vi "Animacion2.vi"() -> ()   [LabVIEW 2017]
uses:
  <vilib>/picture/picture.llb/Draw True-Color Pixmap.vi
panel:
  in  "Donde?":cluster{"x":i16, "y":i16}
  out "Mundo":picture
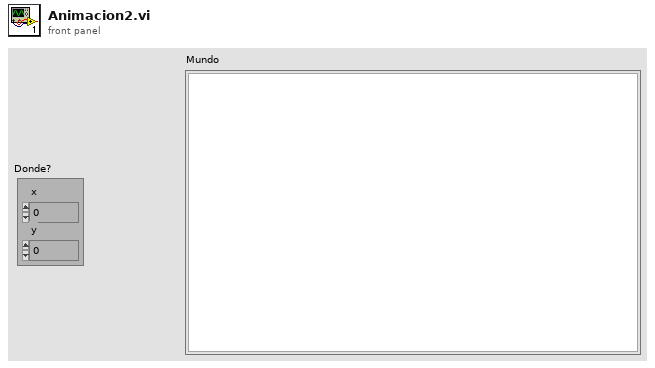
[diagram p1: front panel]
types:
  T1 = typedef "imagedata.ctl" = cluster{"image type":i32, "image depth":i32, "image":u8[], "mask":u8[], "colors":u32[], "Rectangle":cluster{"left":i16, "top":i16, "right":i16, "bottom":i16}}
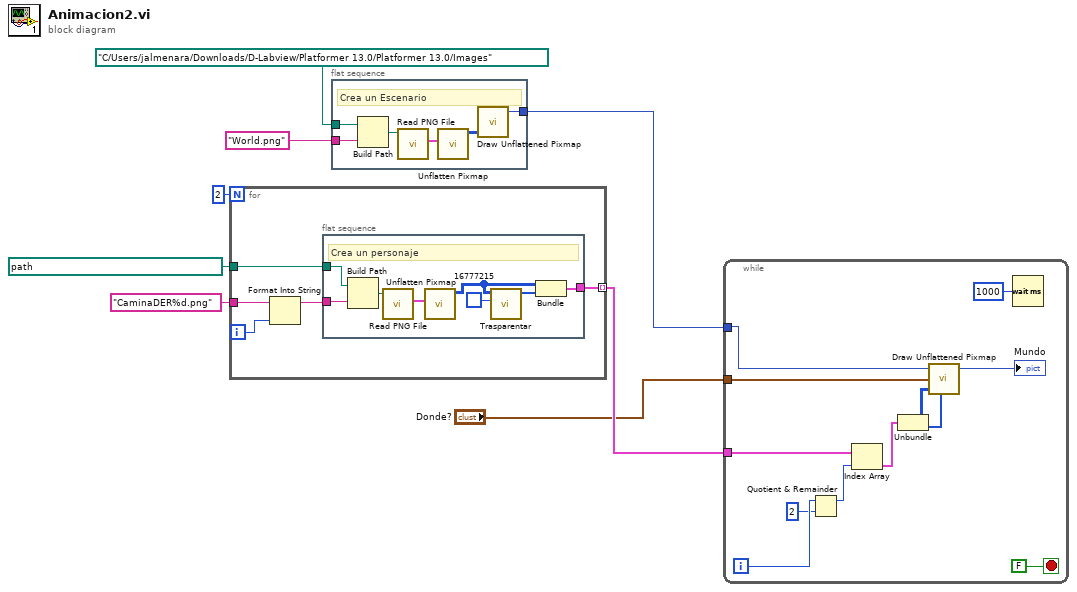
[diagram p0: block diagram]
diagram:
  n1 = for {
    N: 2 -> [_]
    tunnel: [w13] -> w5 mode=indexing
    tunnel: path "F:/Prog/LabVIEW/Pruebas/Animación" ("path to PNG file") -> [w10]
    tunnel: "CaminaDER%d.png" ("format string") -> [w9]
    i -> [w12]
    n2 = Format Into String(format string=w9, w12) -> (resulting string=w11:string)  [unwired: 2 in, 1 out]
    n3 = flat-sequence {
      tunnel: w11 -> [w21]
      tunnel: [w15] -> w13
      tunnel: w10 -> [w14]
      frame #0 {
        # "Crea un personaje"
        n4 = Build Path(base path=w14, name or relative path=w21) -> (appended path=w20:path)
        n5 = call <vilib>:"Read PNG File.vi"("path to PNG file"=w20) -> ("image data"=w19:T1)  [unwired: 8 in, 2 out]
        n6 = call <vilib>:"Unflatten Pixmap.vi"("image data"=w19) -> ("24-bit pixmap"=w17:u32[][])  [unwired: 4 in, 6 out]
        n7 = call "Trasparentar.vi"("Background Color"=u32 16777215, "24-bit pixmap"=w17) -> ("Mask"=w16:u8[])  [unwired: 9 in]
        n8 = Bundle("24-bit pixmap"=w17, "Mask"=w16) -> (w15:cluster{"24-bit pixmap":u32[][], "Mask":u8[]})  [unwired: 1 in]
      }
    }
  }
  n9 = flat-sequence {
    tunnel: "World.png" ("format string") -> [w26]
    tunnel: path "C:/Users/jalmenara/Downloads/D-Labview/Platformer 13.0/Platformer 13.0/Images" ("path to PNG file") -> [w25]
    tunnel: [w22] -> w3
    frame #0 {
      # "Crea un Escenario"
      n10 = Build Path(base path=w25, name or relative path=w26) -> (appended path=w24:path)
      n11 = call <vilib>:"Read PNG File.vi"("path to PNG file"=w24) -> ("image data"=w27:T1)  [unwired: 8 in, 2 out]
      n12 = call <vilib>:"Unflatten Pixmap.vi"("image data"=w27) -> ("24-bit pixmap"=w23:u32[][])  [unwired: 4 in, 6 out]
      n13 = call-poly <vilib>:"Draw Unflattened Pixmap.vi"("data (RGB format)"=w23) -> ("new picture"=w22:picture)  [unwired: 8 in]
    }
  }
  n14 = while {
    tunnel: w5 -> [w36]
    tunnel: "Donde?" -> [w32]
    tunnel: w3 -> [w28]
    i -> [w39]
    stop <- FALSE stop-if-true
    n15 = Quotient & Remainder(x=w39, y=2) -> (x-y*floor(x/y)=w37:i32)  [unwired: 1 out]
    n16 = Index Array(array=w36, index=w37) -> (element=w35:cluster{"24-bit pixmap":u32[][], "Mask":u8[]})
    n17 = Unbundle(w35) -> ("24-bit pixmap"=w34:u32[][], "Mask"=w33:u8[])
    n18 = call-poly <vilib>:"Draw Unflattened Pixmap.vi"("picture"=w28, "top left point(0, 0)"=w32, "data (RGB format)"=w34, "mask"=w33) -> ("new picture"=→"Mundo":picture)  [unwired: 5 in]
    n19 = Wait (ms)(milliseconds to wait=u32 1000) -> ()  [unwired: 1 out]
  }
